vi "TLPM RecordData.vi"(5 "BaseDataPath":path, 7 "Power In":dbl, 8 "error in (no error)":errorcluster caption="entrée d'erreur (pas d'erreur)", 9 "StartTimeIn":dbl, 10 "PwIdxIn":i32, 11 "PowerDataIn":dbl[](array[numeric])) -> (0 "error out":errorcluster caption="sortie d'erreur", 1 "StartTime":dbl, 2 "PwIdxOut":i32, 3 "PowerData":dbl[](array[numeric]))   [LabVIEW 2019]
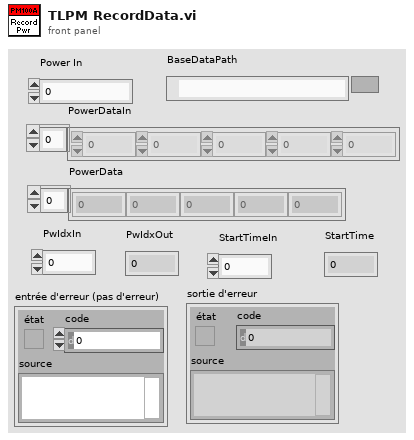
[diagram p1: front panel]
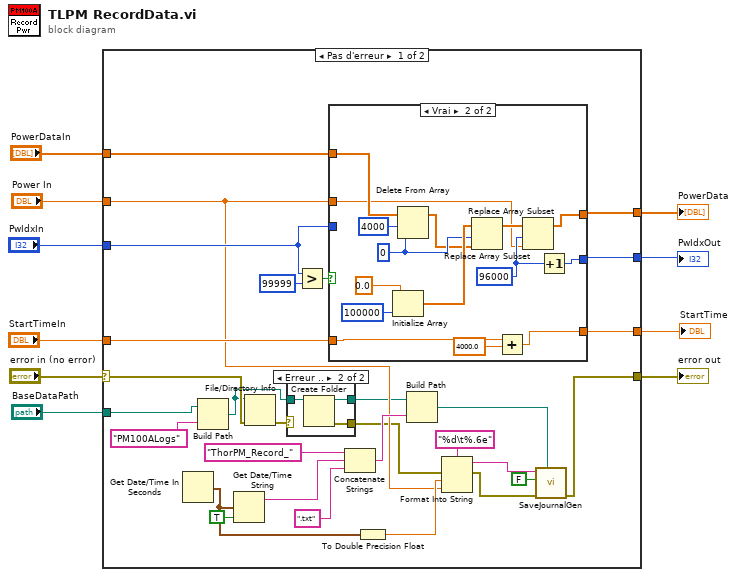
[diagram p0: block diagram]
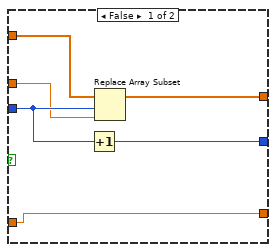
[diagram p3: hidden frame]
diagram:
  n1 = case shown="Pas d'erreur" "error in (no error)" {
    selector: "error in (no error)" -> [w15 w66]
    tunnel: [w39 _] -> w10
    tunnel: "PowerDataIn" -> [w38 _]
    tunnel: "PwIdxIn" -> [w37 _]
    tunnel: [w34 _] -> w7
    tunnel: [w19 w66] -> w5
    tunnel: "StartTimeIn" -> [w33 _]
    tunnel: "Power In" -> [w20 _]
    tunnel: [w32 _] -> w2
    tunnel: "BaseDataPath" -> [w17 _]
    frame No Error {
      n2 = Get Date/Time In Seconds() -> (seconds since 1Jan1904=w23:timestamp)
      n3 = Build Path(base path=w17, name or relative path="PM100ALogs" ("nom ou chemin relatif")) -> (appended path=w13:path)
      n4 = Get Date/Time String(seconds (now)=w23, want seconds? (F)=TRUE ("secondes ? (F)")) -> (date string=w29:string)  [unwired: 1 in, 1 out]
      n5 = File/Directory Info(path=w13, error in=w15) -> (error out=w14:errorcluster)  [unwired: 6 out]
      n6 = case shown="Erreur .." w14 {
        selector: w14 -> [w41 _]
        tunnel: w13 -> [w40 w44]
        tunnel: [w41 w43] -> w12
        tunnel: [w40 w42] -> w11
        frame No Error {
        }
        frame Error {
          n7 = Create Folder(path (use dialog)=w44) -> (created path=w42:path, error out=w43:errorcluster)  [unwired: 2 in, 1 out]
        }
      }
      n8 = Greater?(x=w37, y=99999) -> (0:w35:bool)
      n9 = case shown="Vrai" w35 {
        tunnel: [w50 w57] -> w39
        tunnel: w38 -> [w49 w65]
        tunnel: w37 -> [w48 _]
        tunnel: [w47 w55] -> w34
        tunnel: w33 -> [w45 w53]
        tunnel: w20 -> [w46 w54]
        tunnel: [w45 w51] -> w32
        frame False {
          n10 = Increment(x=w48) -> (x+1=w47:i32)
          n11 = Replace Array Subset(array=w49, new element=w46, index=w48) -> (w50:dbl[])
        }
        frame True {
          w56 = 96000 ("y")
          w60 = 0 ("indice")
          n12 = Initialize Array(0.0 ("élément"), 100000 ("taille de la dimension")) -> (w62:dbl[])
          n13 = Delete From Array(array=w65, length=4000 ("longueur"), index=w60) -> (array with subset deleted=w59:dbl[])  [unwired: 1 out]
          n14 = Replace Array Subset(array=w62, new element=w59, index=w60) -> (w58:dbl[])
          n15 = Add(x=w53, y=4000.0) -> (x+y=w51:dbl)
          n16 = Replace Array Subset(array=w58, new element=w54, index=w56) -> (w57:dbl[])
          n17 = Increment(x=w56) -> (x+1=w55:i32)
        }
      }
      n18 = Concatenate Strings("ThorPM_Record_" ("chaîne"), w29, ".txt" ("chaîne")) -> (w30:string)
      n19 = To Double Precision Float(number=w23) -> (double precision float=w21:dbl)
      n20 = Build Path(base path=w11, name or relative path=w30) -> (appended path=w18:path)
      n21 = Format Into String(format string="%d\t%.6e" ("chaîne de format"), error in=w12, w21, w20) -> (resulting string=w25:string, error out=w26:errorcluster)  [unwired: 1 in]
      n22 = call <userlib>:"SaveJournalGen.vi"("CheminSauv"=w18, "error in"=w26, "Include Date_Time"=FALSE, "Journal Text"=w25) -> ("error out"=w19:errorcluster)  [unwired: 6 in, 1 out]
    }
    frame Error {
    }
  }
  "PowerData" <- w10
  "PwIdxOut" <- w7
  "error out" <- w5
  "StartTime" <- w2
